vi "ParseDocString.vi"(11 "docstring":string) -> (1 "outputs":string, 2 "inputs":string, 3 "function name":string)   [LabVIEW 2014, in "Python Functions.lvlib"]
uses:
  Python Functions.lvlib
  <vilib>/regexp/Match Regular Expression.xnode
panel:
  out "error out":errorcluster
  in  "error in":errorcluster
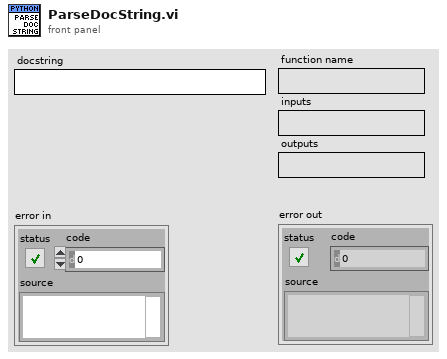
[diagram p1: front panel]
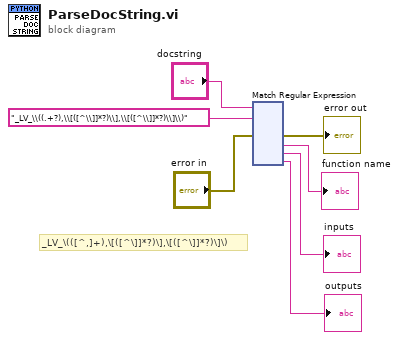
[diagram p0: block diagram]
diagram:
  # "_LV_\\(([^,]+),\\[([^\\]]*?)\\],\\[([^\\]]*?)\\]\\)"
  n1 = xnode "Match Regular Expression"("input string"="docstring", "regular expression"="_LV_\\((.+?),\\[([^\\]]*?)\\],\\[([^\\]]*?)\\]\\)" ("format string"), "error in"="error in") -> ("error out"=→"error out":errorcluster, "submatch 1"=→"function name":string, "submatch 2"=→"inputs":string, "submatch 3"=→"outputs":string)  [unwired: 3 in, 4 out]
